vi "SV TDMS Write Spectrum (N Ch).vi"(0 "tdms file":refnum<k34>, 5 "group name in":string="Spectrum", 7 "channel names in":string[](array[string]), 9 "spectra":cluster{"x0":dbl, "dx":dbl, "array":dbl[]}[](array[cluster]), 11 "error in":errorcluster, 12 "component":T1=32 items=["Magnitude"=32, "Phase"=33, "Real"=34, "Imaginary"=35, "Complex"=345, "Coherence"=36, "Unknown"=99], 13 "spectra info":T2[](array[typedef]) {"x-axis units" items=["Time (s)"=0, "Frequency-CB (Hz)"=1, "Frequency-CPB (Hz)"=1248, "Frequency-Arbitrary (Hz)"=2357, "Quefrency (s)"=2, "Revolutions (rev)"=3, "Order"=4, "Speed (RPM)"=11, "Speed (rad/s)"=21, "Index"=65535]; "weighting filter" items=["Linear", "A-weighting", "B-weighting", "C-weighting", "ITU-R 468-4", "Dolby", "CCITT", "C-message", "Wb", "Wc", "Wd", "We", "Wf", "Wh", "Wj", "Wk", "Wm", "AES17 20 kHz lowpass", "AES17 40 kHz lowpass", "AES17 20 kHz highpass", "AES17 40 kHz highpass"]; "dB reference [EU]" format="%.2f"; "engineering units" items=["custom..."=0, "V"=1, "A"=21, "C"=30, "pC"=31, "s"=32, "-"=29, "Pa"=2, "N"=20, "g"=3, "m/s^2"=4, "m/s"=5, "m"=6, "mm/s"=12, "mm"=13, "micron/s"=14, "micron"=15, "in/s^2"=7, "in/s"=8, "in"=9, "mil/s"=10, "mil"=11, "rad/s^2"=16, "rad/s"=17, "rad"=18, "deg/s^2"=26, "deg/s"=27, "deg"=28, "RPM"=22, "cycle/s^2"=23, "Hz"=24, "cycle"=25, "strain"=19]; "spectral info"."window" items=["None "=0, "Hanning"=1, "Hamming"=2, "Blackman-Harris"=3, "Exact Blackman"=4, "Blackman"=5, "Flat Top"=6, "4 Term B-Harris "=7, "7 Term B-Harris"=8, "Low Sidelobe"=9, "Force - Exponential"=10, "Gaussian"=62]}) -> (4 "tdms file out":refnum<k34>, 6 "group name out":string, 8 "channel names out":string[](array[string]), 15 "error out":errorcluster)   [LabVIEW 2017]
doc: "Writes data to the specified .tdms file in a format specific to the polymorphic instance. Wire data to the <B>scaled signal [EU]</B> input to determine the polymorphic instance to use or manually select the instance."
uses:
  <vilib>/addons/_NISVFA/_Shared subVIs/Controls/svc_Spectrum Info.ctl
  <vilib>/addons/_NISVFA/_Shared subVIs/Controls/svc_X-Axis Units.ctl
  <vilib>/addons/_NISVFA/_Shared subVIs/Controls/svc_Spectrum Type.ctl
  <vilib>/addons/_NISVFA/_Shared subVIs/Controls/svc_Engineering Units Text Ring.ctl
  <vilib>/addons/_NISVFA/_Shared subVIs/Controls/svc_Weighting Filter Text Ring.ctl
  <vilib>/addons/_NISVFA/_Shared subVIs/Controls/svc_Complimentary Spectrum Units.ctl
  <vilib>/addons/_NISVFA/_Shared subVIs/Controls/NI Spectrum Component.ctl
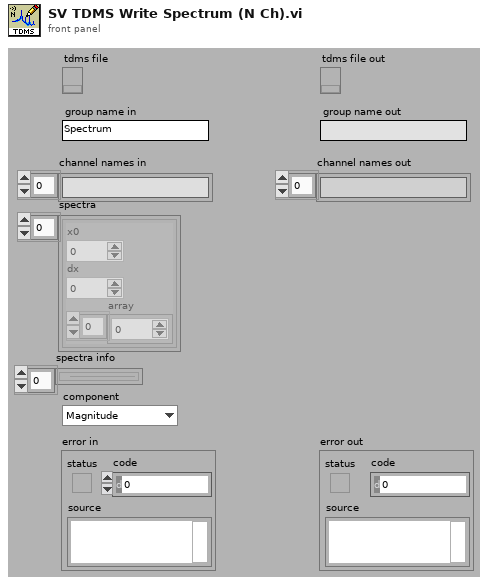
[diagram p1: front panel]
types:
  T1 = typedef "NI Spectrum Component.ctl" = u16
  T2 = typedef "svc_Spectrum Info.ctl" = cluster{"channel name":string, "description":string, "x-axis units":T3, "spectral info":cluster{"spectrum type":T4, "linear/dB":enum16{"linear", "dB"}, "window":u16, "window size":i32, "FFT size":i32}, "engineering units":T5, "custom label":string, "dB reference [EU]":dbl, "peak units":enum16{"rms", "peak", "peak-peak"}, "weighting filter":T6, "spectral density?":bool, "unit label":string, "spectrum skewed?":bool, "complimentary spectrum units":T7}
  T3 = typedef "svc_X-Axis Units.ctl" = u16
  T4 = typedef "svc_Spectrum Type.ctl" = enum16{"FFT Spectrum [complex]", "Amplitude [Magnitude]", "Power [Magnitude^2]", "Cross Spectrum [complex]", "Frequency Response [Complex]"}
  T5 = typedef "svc_Engineering Units Text Ring.ctl" = u16
  T6 = typedef "svc_Weighting Filter Text Ring.ctl" = u16
  T7 = typedef "svc_Complimentary Spectrum Units.ctl" = enum16{"none", "radians", "degrees", "cycles", "imaginary"}
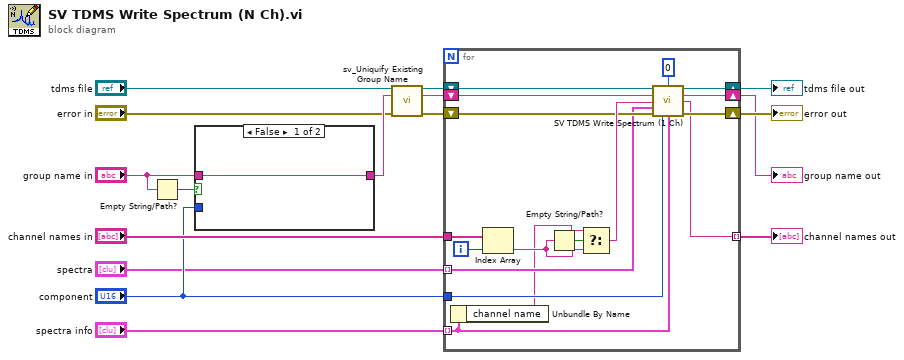
[diagram p0: block diagram]
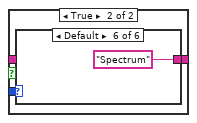
[diagram p2: hidden frame]
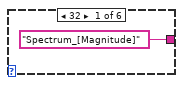
[diagram p3: hidden frame]
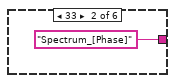
[diagram p4: hidden frame]
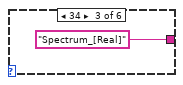
[diagram p5: hidden frame]
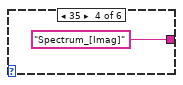
[diagram p6: hidden frame]
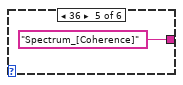
[diagram p7: hidden frame]
diagram:
  n1 = Empty String/Path?(string/path="group name in") -> (empty?=w13:bool)
  n2 = case shown="False" w13 {
    tunnel: "component" -> [_ w19]
    tunnel: [w17 w18] -> w4
    tunnel: "group name in" -> [w17 _]
    frame False {
    }
    frame True {
      n3 = case shown="Default" w19 {
        tunnel: ["Spectrum_[Magnitude]" "Spectrum_[Phase]" "Spectrum_[Real]" "Spectrum_[Imag]" "Spectrum_[Coherence]" "Spectrum"] -> w18
        frame 32 {
        }
        frame 33 {
        }
        frame 34 {
        }
        frame 35 {
        }
        frame 36 {
        }
        frame Default {
        }
      }
    }
  }
  n4 = call <vilib>:"sv_Uniquify Existing Group Name.vi"("tdms file ref"="tdms file", "group name"=w4, "error in"="error in") -> ("tdms file out"=w5:refnum<k34>, "unique group"=w3:string, "error out"=w1:errorcluster)  [unwired: 10 in]
  n5 = for {
    tunnel: "channel names in" -> [w40]
    tunnel: "spectra info" -> [w27] mode=indexing
    tunnel: "component" -> [w30]
    tunnel: "spectra" -> [w31] mode=indexing
    tunnel: [w32] -> w7 mode=indexing
    shift-right: [w34] -> w10
    shift-left: w5 -> [w39]
    shift-right: [w35] -> w11
    shift-left: w1 -> [w36]
    shift-right: [w33] -> w8
    shift-left: w3 -> [w38]
    i -> [w41]
    n6 = Unbundle By Name(w27) -> ("channel name"=w28:string)
    n7 = Index Array(array=w40, index=w41) -> (element=w29:string)
    n8 = Empty String/Path?(string/path=w29) -> (empty?=w42:bool)
    n9 = Select(t=w28, s=w42, f=w29) -> (s? t:f=w37:string)
    n10 = call <vilib>:"SV TDMS Write Spectrum (1 Ch).vi"("tdms file"=w39, "write mode"=i16 0, "group name in"=w38, "channel name in"=w37, "spectrum"=w31, "error in"=w36, "component"=w30, "spectrum info"=w27) -> ("tdms file out"=w34:refnum<k34>, "group name out"=w33:string, "channel name out"=w32:string, "error out"=w35:errorcluster)  [unwired: 4 in]
  }
  "error out" <- w11
  "tdms file out" <- w10
  "group name out" <- w8
  "channel names out" <- w7
